vi "Get Name.vi"(7 "Tree ID":string, 8 "Error In":errorcluster, 11 "Tree Manager":refnum<data-value>) -> (0 "Error Out":errorcluster, 1 "Name":string, 3 "Tree Manager":refnum<data-value>)   [LabVIEW 2017, in "Tree API.lvlib" / "Tree.lvclass"]
doc: "Get the Name of the Tree."
uses:
  Tree.lvclass
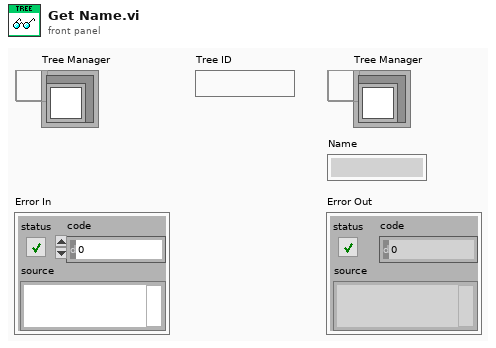
[diagram p1: front panel]
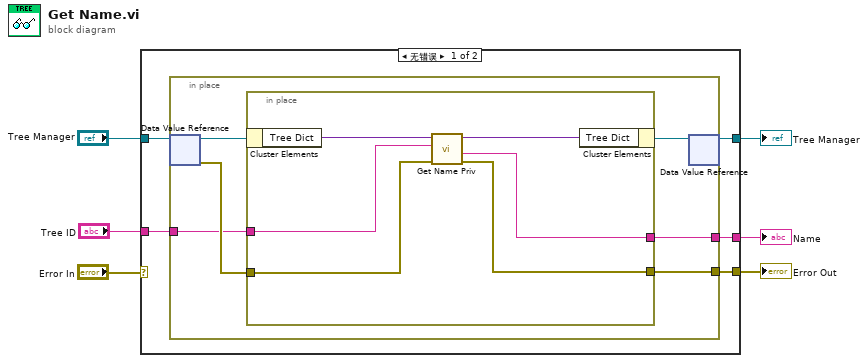
[diagram p0: block diagram]
diagram:
  n1 = case shown="无错误" "Error In" {
    selector: "Error In" -> [_ w24]
    tunnel: "Tree Manager" -> [w11 w25]
    tunnel: [w10 w25] -> w5
    tunnel: [w9 w24] -> w3
    tunnel: "Tree ID" -> [w8 _]
    tunnel: [w7 _] -> w1
    frame No Error {
      n2 = in-place {
        in-place-border: [w16] -> w9
        in-place-border: w8 -> [w13]
        in-place-border: [w12] -> w7
        n3 = in-place-dvr #1(w11) -> (w17:refnum<class "Tree.lvclass">, w14:errorcluster)
        n4 = in-place {
          in-place-border: [w20] -> w16
          in-place-border: w14 -> [w21]
          in-place-border: w13 -> [w19]
          in-place-border: [w18] -> w12
          n5 = in-place-cluster #2(w17) -> ("Tree Dict"=w23:variant)
          n6 = call "Get Name Priv.vi"("error in"=w21, "Unique ID"=w19, "Tree Dictionary"=w23) -> ("error out"=w20:errorcluster, "Name"=w18:string, "Tree Dictionary Out"=w22:variant)  [unwired: 6 in]
          n7 = in-place-cluster #2("Tree Dict"=w22) -> (w15:refnum<class "Tree.lvclass">)
        }
        n8 = in-place-dvr #1(w15) -> (w10:refnum<data-value>)  [unwired: 1 out]
      }
    }
    frame Error {
    }
  }
  "Tree Manager" <- w5
  "Error Out" <- w3
  "Name" <- w1
